vi "Ping N Times.vi"(8 "error in (no error)":errorcluster, 10 "Ping Test":T1, 11 "Network Test in":refnum<class "Network Test.lvclass">) -> (0 "error out":errorcluster, 3 "Network Test out":refnum<class "Network Test.lvclass">)   [LabVIEW 2017, in "Network Test.lvlib" / "Network Test.lvclass"]
uses:
  Network Test.lvclass
  Ping Test Configuration.ctl
  <vilib>/Utility/miscctls.llb/LVRowAndColumnTypeDef.ctl
  Network Test.lvclass/Network Test.ctl
  Network Test.lvlib
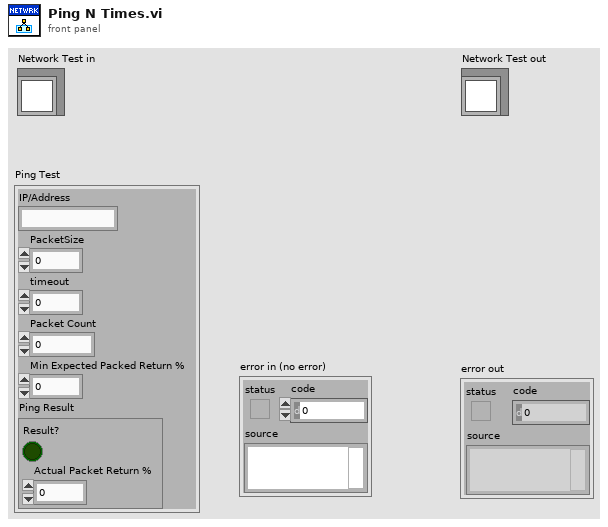
[diagram p1: front panel]
types:
  T1 = typedef "Network Test.lvlib/Ping Test Configuration.ctl" = cluster{"IP/Address":string, "PacketSize":i32, "timeout":i32, "Packet Count":i32, "Min Expected Packed Return %":dbl, "Ping Result":cluster{"Result?":bool, "Actual Packet Return %":dbl}}
  T2 = typedef "LVRowAndColumnTypeDef.ctl" = cluster{"Row":i32, "Column":i32}
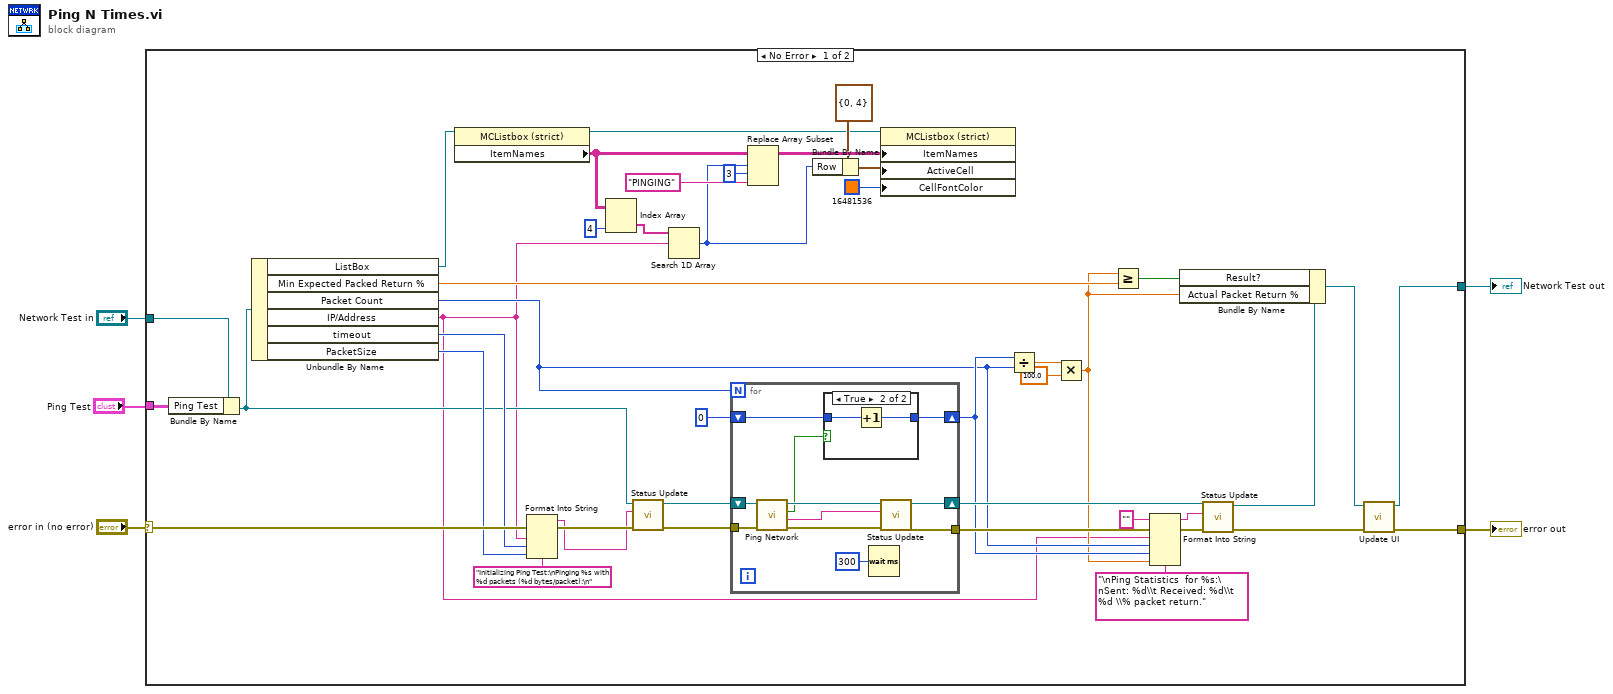
[diagram p0: block diagram]
diagram:
  n1 = case shown="No Error" "error in (no error)" {
    selector: "error in (no error)" -> [w47 w64]
    tunnel: [w23 w64] -> w4
    tunnel: [w22 w63] -> w2
    tunnel: "Network Test in" -> [w20 w63]
    tunnel: "Ping Test" -> [w21 _]
    frame No Error {
      n2 = Bundle By Name(cluster=w20, "Ping Test"=w21) -> (w19:refnum<class "Network Test.lvclass">)
      n3 = Unbundle By Name(w19) -> ("ListBox"=w18:refnum<vi>, "Min Expected Packed Return %"=w29:dbl, "Packet Count"=w30:i32, "IP/Address"=w15:string, "timeout"=w45:i32, "PacketSize"=w46:i32)
      n4 = property class="MCListbox (strict)"(reference=w18) -> (reference out=w6:refnum<vi>, "ItemNames"=w14:string[][])  [unwired: 1 in, 1 out]
      n5 = Format Into String(format string="Initializing Ping Test:\nPinging %s with  %d packets (%d bytes/packet):\n", error in=w47, w15, w45, w46) -> (resulting string=w40:string, error out=w43:errorcluster)  [unwired: 1 in]
      n6 = Index Array(array=w14, index (col)=4 ("disabled index (col)")) -> (element=w16:string[])  [unwired: 1 in]
      n7 = call-dynamic "Status Update.vi"("error in (no error)"=w43, "Status"=w40, "Network Test in"=w19) -> ("error out"=w42:errorcluster, "Network Test out"=w41:refnum<class "Network Test.lvclass">)  [unwired: 7 in]
      n8 = Search 1D Array(1D array=w16, element=w15) -> (index of element=w8:i32)  [unwired: 1 in]
      n9 = for {
        N: w30 -> [_]
        tunnel: w42 -> [w59]
        tunnel: [w56] -> w35
        shift-right: [w54] -> w37
        shift-left: w41 -> [w58]
        shift-right: [w51] -> w31
        shift-left: 0 -> [w52]
        n10 = call "Ping Network.vi"("error in (no error)"=w59, "Network Test in"=w58) -> ("error out"=w57:errorcluster, "Response"=w53:string, "PingSuccess?"=w50:bool, "Network Test out"=w55:refnum<class "Network Test.lvclass">)  [unwired: 6 in]
        n11 = case shown="True" w50 {
          tunnel: w52 -> [w60 w62]
          tunnel: [w60 w61] -> w51
          frame False {
          }
          frame True {
            n12 = Increment(x=w62) -> (x+1=w61:i32)
          }
        }
        n13 = Wait (ms)(milliseconds to wait=u32 300) -> ()  [unwired: 1 out]
        n14 = call-dynamic "Status Update.vi"("error in (no error)"=w57, "Status"=w53, "Network Test in"=w55) -> ("error out"=w56:errorcluster, "Network Test out"=w54:refnum<class "Network Test.lvclass">)  [unwired: 7 in]
      }
      n15 = Replace Array Subset(array=w14, new element="PINGING" ("new element/subarray"), index (row)=w8, index (col)=3 ("disabled index (col)")) -> (w11:string[][])
      n16 = Bundle By Name(cluster=T2 {"Row"=0, "Column"=4} ("Active Cell:Active Cell"), "Row"=w8) -> (w9:T2)
      n17 = property class="MCListbox (strict)"(reference=w6, "ItemNames"=w11, "ActiveCell"=w9, "CellFontColor"=u32 16481536) -> ()  [unwired: 1 in, 2 out]
      n18 = Divide(x=w31, y=w30) -> (x/y=w33:dbl)
      n19 = Multiply(x=w33, y=100.0) -> (x*y=w27:dbl)
      n20 = Greater Or Equal?(x=w27, y=w29) -> (x >= y?=w28:bool)
      n21 = Format Into String(format string="\nPing Statistics  for %s:\nSent: %d\\t Received: %d\\t %d \\% packet return.", initial string="", error in=w35, w15, w30, w31, w27) -> (resulting string=w36:string, error out=w34:errorcluster)
      n22 = call-dynamic "Status Update.vi"("error in (no error)"=w34, "Status"=w36, "Network Test in"=w37) -> ("error out"=w24:errorcluster, "Network Test out"=w26:refnum<class "Network Test.lvclass">)  [unwired: 7 in]
      n23 = Bundle By Name(cluster=w26, "Result?"=w28, "Actual Packet Return %"=w27) -> (w25:refnum<class "Network Test.lvclass">)
      n24 = call "Update UI.vi"("error in (no error)"=w24, "Network Test in"=w25) -> ("error out"=w23:errorcluster, "Network Test out"=w22:refnum<class "Network Test.lvclass">)  [unwired: 8 in]
    }
    frame Error {
    }
  }
  "error out" <- w4
  "Network Test out" <- w2
